vi "main_GBATP_Portain_Sample.vi"() -> ()   [LabVIEW 2020]
panel:
  out "Even Number":dbl=1.0
  out "X, Y, Z, S":i32=3
  out "Value":string="0"
  out "Index 2":i32=95
  out "Index":i32=95
  out "Current Position(mm) 2":dbl
  in  "Occupied Length by Air(mm)  2":dbl format="%#_13g"
  out "Value 2":string="0"
  out "X, Y, Z, S 2":i32=3
  out "Index 4":i32=123
  out "Index 3":i32=123
  in  "Stop Button":bool
  in  "ATP":bool=TRUE
  out "ATP":bool=TRUE
  out "Sample":bool=TRUE
  in  "Occupied Length by Air(mm)  3":dbl format="%#_13g"
  out "Current Position(mm) 3":dbl
  out "ATPPortain":bool=TRUE
  out "X, Y, Z, S 3":i32=3
  out "Index 6":i32=95
  out "Value 3":string="0"
  out "Index 5":i32=95
  in  "Setting Tab":T1(tab)
  out "all rows":string[][](array[string])=[["58"], ["257"], ["0"], ["0"], ["58"], ["257"], ["100"], ["50"], ["58"], ["257"], ["0"], ["50"], ["58"], ["470"], ["0"], ["50"], ["58"], ["470"], ["100"], ["0"], ["58"], ["470"], ["0"], ["0"], ["120"], ["470"], ["0"], ["0"], ["120"], ["470"], ["100"], ["50"], ["120"], ["470"], ["0"], ["50"], ["120"], ["550"], ["0"], ["50"], ["120"], ["550"], ["100"], ["0"], ["120"], ["550"], ["0"], ["0"], ["120"], ["470"], ["0"], ["0"], ["120"], ["470"], ["100"], ["50"], ["120"], ["470"], ["0"], ["50"], ["120"], ["550"], ["0"], ["50"], ["120"], ["550"], ["100"], ["0"], ["120"], ["550"], ["0"], ["0"], ["120"], ["470"], ["0"], ["0"], ["120"], ["470"], ["100"], ["50"], ["120"], ["470"], ["0"], ["50"], ["120"], ["550"], ["0"], ["50"], ["120"], ["550"], ["100"], ["0"], ["120"], ["550"], ["0"], ["0"]]
  in  "format (%.3f)":string="%.3f"
  in  "transpose (no:F)":bool
  in  "type (empty)":string[][](array[string])
  in  "delimiter (Tab)":string="\t"
  out "Size(s)":i32=96
  in  "Sampling Measurement Time(S)":dbl=10.0
  out "Current Position(mm)":dbl
  in  "Occupied Length by Air(mm)":dbl format="%#_13g"
  out "Action":bool=TRUE
  out "Current Time Index":i32=10
  in  "file path (dialog if empty)":path=path "C:/Users/user/Desktop/AutoSampler/AutoSampler _GB/ATP.txt"
  in  "start of read offset (chars.:0)":i32
  in  "max characters/row  (no limit:0)":i32
  out "mark after read (chars.)":i32=406
  in  "number of rows (all:-1)":i32=-1
  out "EOF?":bool
  out "mark after read (chars.) 2":i32=1632
  out "all rows 2":string[][](array[string])=[["58"], ["257"], ["0"], ["0"], ["58"], ["257"], ["100"], ["0"], ["58"], ["257"], ["0"], ["0"], ["58"], ["0"], ["0"], ["0"], ["58"], ["0"], ["100"], ["0"], ["58"], ["0"], ["0"], ["0"], ["120"], ["470"], ["0"], ["0"], ["120"], ["470"], ["100"], ["0"], ["120"], ["470"], ["0"], ["0"], ["120"], ["550"], ["0"], ["0"], ["120"], ["550"], ["100"], ["0"], ["120"], ["550"], ["0"], ["0"], ["120"], ["470"], ["0"], ["0"], ["120"], ["470"], ["100"], ["0"], ["120"], ["470"], ["0"], ["0"], ["120"], ["550"], ["0"], ["0"], ["120"], ["550"], ["100"], ["0"], ["120"], ["550"], ["0"], ["0"], ["120"], ["470"], ["0"], ["0"], ["120"], ["470"], ["100"], ["0"], ["120"], ["470"], ["0"], ["0"], ["120"], ["550"], ["0"], ["0"], ["120"], ["550"], ["100"], ["0"], ["120"], ["550"], ["0"], ["0"], ["58"], ["257"], ["0"], ["0"], ["58"], ["257"], ["100"], ["0"], ["58"], ["257"], ["0"], ["0"], ["58"], ["9"], ["0"], ["0"], ["58"], ["9"], ["100"], ["0"], ["58"], ["9"], ["0"], ["0"], ["120"], ["470"], ["0"], ["0"], ["120"], ["470"], ["100"], ["0"], ["120"], ["470"], ["0"], ["0"], ["120"], ["550"], ["0"], ["0"], ["120"], ["550"], ["100"], ["0"], ["120"], ["550"], ["0"], ["0"], ["120"], ["470"], ["0"], ["0"], ["120"], ["470"], ["100"], ["0"], ["120"], ["470"], ["0"], ["0"], ["120"], ["550"], ["0"], ["0"], ["120"], ["550"], ["100"], ["0"], ["120"], ["550"], ["0"], ["0"]]
  in  "format (%.3f) 2":string="%.3f"
  in  "transpose (no:F) 2":bool
  in  "type (empty) 2":string[][](array[string])
  in  "delimiter (Tab) 2":string="\t"
  out "EOF? 2":bool
  out "Sample Size(s) 2":i32=168
  in  "file path (dialog if empty) 4":path=path "C:/Users/user/Desktop/AutoSampler/AutoSampler _GB/SamplePosition.txt"
  in  "start of read offset (chars.:0) 2":i32
  in  "max characters/row  (no limit:0) 2":i32
  in  "number of rows (all:-1) 2":i32=-1
  in  "file path (dialog if empty) 3":path=path "C:/Users/user/Desktop/AutoSampler/AutoSampler _GB/ProteinPosition.txt"
  out "mark after read (chars.) 3":i32=1632
  out "all rows 3":string[][](array[string])=[["58"], ["63"], ["0"], ["0"], ["58"], ["63"], ["100"], ["0"], ["58"], ["63"], ["0"], ["0"], ["58"], ["257"], ["0"], ["0"], ["58"], ["257"], ["100"], ["0"], ["58"], ["257"], ["0"], ["0"], ["120"], ["470"], ["0"], ["0"], ["120"], ["470"], ["100"], ["0"], ["120"], ["470"], ["0"], ["0"], ["120"], ["550"], ["0"], ["0"], ["120"], ["550"], ["100"], ["0"], ["120"], ["550"], ["0"], ["0"], ["120"], ["470"], ["0"], ["0"], ["120"], ["470"], ["100"], ["0"], ["120"], ["470"], ["0"], ["0"], ["120"], ["550"], ["0"], ["0"], ["120"], ["550"], ["100"], ["0"], ["120"], ["550"], ["0"], ["0"], ["120"], ["470"], ["0"], ["0"], ["120"], ["470"], ["100"], ["0"], ["120"], ["470"], ["0"], ["0"], ["120"], ["550"], ["0"], ["0"], ["120"], ["550"], ["100"], ["0"], ["120"], ["550"], ["0"], ["0"]]
  in  "format (%.3f) 3":string="%.3f"
  in  "transpose (no:F) 3":bool
  in  "type (empty) 3":string[][](array[string])
  in  "delimiter (Tab) 3":string="\t"
  out "EOF? 3":bool
  out "Size(s) 3":i32=96
  in  "start of read offset (chars.:0) 3":i32
  in  "max characters/row  (no limit:0) 3":i32
  in  "number of rows (all:-1) 3":i32=-1
  out "error out":errorcluster={"status"=FALSE, "code"=1073676294, "source"="VISA Read in position_read.vi->main_GBATP_Portain_Sample.vi"}
  out "S Connecting":bool=TRUE
  out "Z Connecting":bool=TRUE
  out "Y Connecting":bool=TRUE
  out "X  Connecting":bool=TRUE
  in  "COM Port":refnum<visa-resource-name>="COM3"
  # "Position :"
  # "(set the Occupied length by Air if the target axis is syringe axis)"
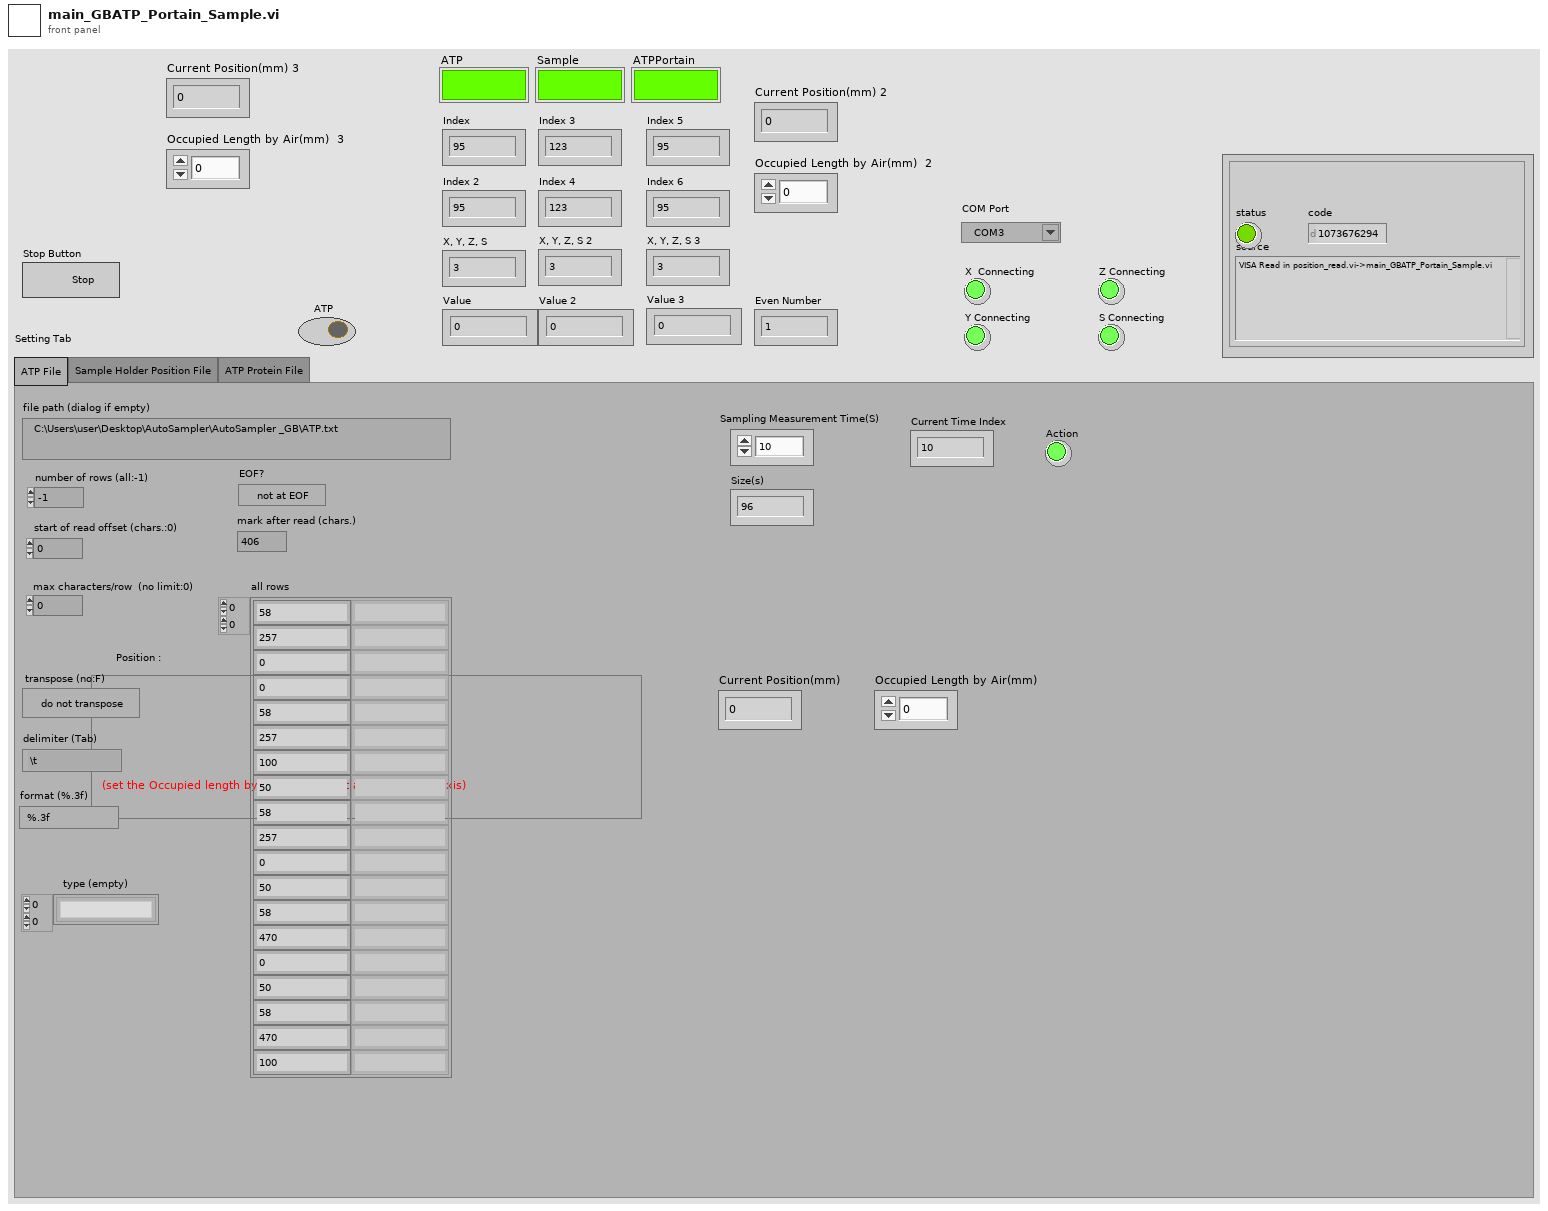
[diagram p1: front panel]
types:
  T1 = enum32{"ATP File", "Sample Holder Position File", "ATP Protein File"}
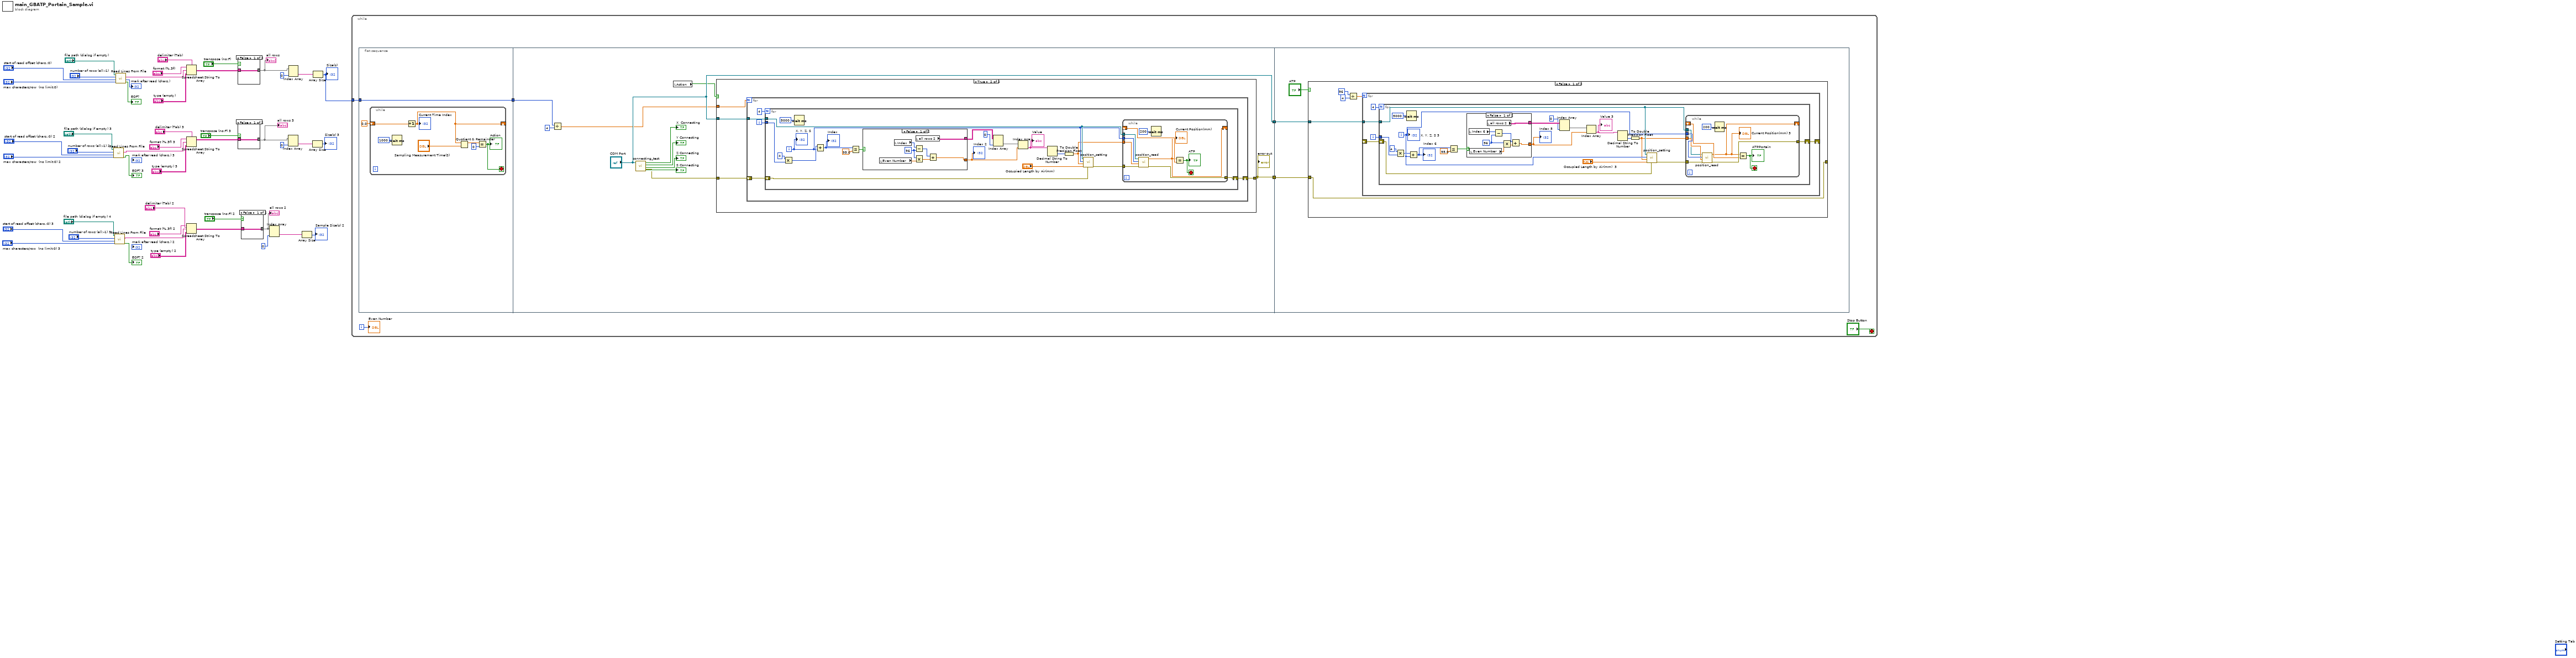
[diagram p0: block diagram]
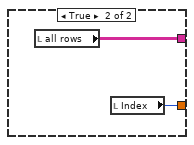
[diagram p3: hidden frame]
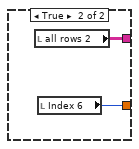
[diagram p4: hidden frame]
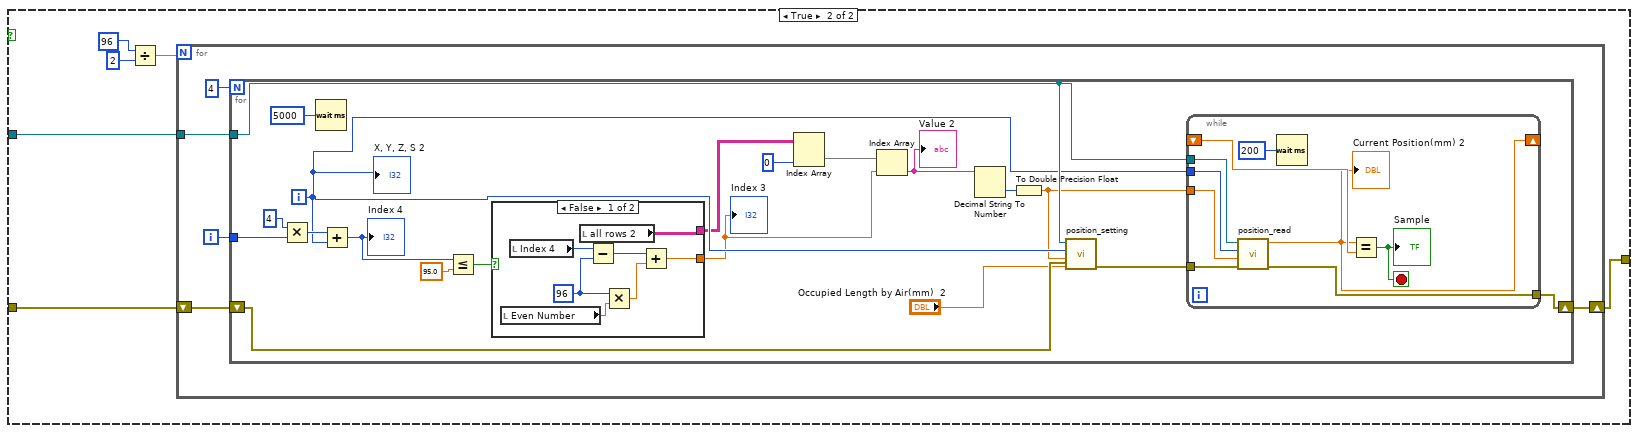
[diagram p5: hidden frame]
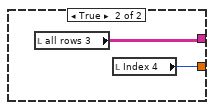
[diagram p6: hidden frame]
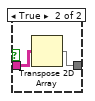
[diagram p7: hidden frame]
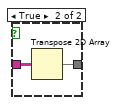
[diagram p8: hidden frame]
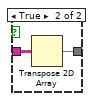
[diagram p9: hidden frame]
diagram:
  n1 = call <vilib>:"Read Lines From File.vi"("file path (dialog if empty)"="file path (dialog if empty) 3", "number of lines (all:-1)"="number of rows (all:-1) 2", "start of read offset (chars.:0)"="start of read offset (chars.:0) 2", "[max characters per line]  (no limit:0)"="max characters/row  (no limit:0) 2") -> ("line string"=w38:string, "EOF?"=→"EOF? 3":bool)  [unwired: 2 in, 2 out]
  n2 = call <vilib>:"Read Lines From File.vi"("file path (dialog if empty)"="file path (dialog if empty) 4", "number of lines (all:-1)"="number of rows (all:-1) 3", "start of read offset (chars.:0)"="start of read offset (chars.:0) 3", "[max characters per line]  (no limit:0)"="max characters/row  (no limit:0) 3") -> ("line string"=w45:string, "EOF?"=→"EOF? 2":bool)  [unwired: 2 in, 2 out]
  n3 = call <vilib>:"Read Lines From File.vi"("file path (dialog if empty)"="file path (dialog if empty)", "number of lines (all:-1)"="number of rows (all:-1)", "start of read offset (chars.:0)"="start of read offset (chars.:0)", "[max characters per line]  (no limit:0)"="max characters/row  (no limit:0)") -> ("line string"=w34:string, "mark after read (chars.)"=→"mark after read (chars.)":i32, "EOF?"=→"EOF?":bool)  [unwired: 2 in, 1 out]
  n4 = Spreadsheet String To Array(delimiter (Tab)="delimiter (Tab)", format string="format (%.3f)", spreadsheet string=w34, array type (2D Dbl)="type (empty)") -> (array=w6:string[][])
  n5 = Spreadsheet String To Array(delimiter (Tab)="delimiter (Tab) 3", format string="format (%.3f) 3", spreadsheet string=w38, array type (2D Dbl)="type (empty) 3") -> (array=w21:string[][])
  n6 = Spreadsheet String To Array(delimiter (Tab)="delimiter (Tab) 2", format string="format (%.3f) 2", spreadsheet string=w45, array type (2D Dbl)="type (empty) 2") -> (array=w12:string[][])
  n7 = case shown="False" "transpose (no:F)" {
    tunnel: [w47 w49] -> w18
    tunnel: w6 -> [w47 w48]
    frame False {
    }
    frame True {
      n8 = Transpose 2D Array(2D array=w48) -> (transposed array=w49:string[][])
    }
  }
  "all rows" <- w18
  n9 = case shown="False" "transpose (no:F) 3" {
    tunnel: [w50 w52] -> w27
    tunnel: w21 -> [w50 w51]
    frame False {
    }
    frame True {
      n10 = Transpose 2D Array(2D array=w51) -> (transposed array=w52:string[][])
    }
  }
  "all rows 3" <- w27
  n11 = case shown="False" "transpose (no:F) 2" {
    tunnel: [w53 w55] -> w19
    tunnel: w12 -> [w53 w54]
    frame False {
    }
    frame True {
      n12 = Transpose 2D Array(2D array=w54) -> (transposed array=w55:string[][])
    }
  }
  "all rows 2" <- w19
  n13 = Index Array "Index Array"(array=w19, index (col)=0) -> (element=w16:string[])  [unwired: 1 in]
  n14 = Index Array "Index Array"(array=w27, index (col)=0) -> (element=w25:string[])  [unwired: 1 in]
  n15 = Index Array "Index Array"(array=w18, index (col)=0) -> (element=w10:string[])  [unwired: 1 in]
  n16 = Array Size(array=w16) -> (size(s)=→"Sample Size(s) 2":i32)
  n17 = Array Size(array=w25) -> (size(s)=→"Size(s) 3":i32)
  n18 = Array Size(array=w10) -> (size(s)=w1:i32)
  "Size(s)" <- w1
  n19 = while {
    tunnel: w1 -> [w58]
    i -> [w56]
    stop <- "Stop Button" stop-if-true
    n20 = flat-sequence {
      tunnel: w58 -> [w63]
      tunnel: [w63] -> w61
      tunnel: [w75] -> w60
      tunnel: ["COM Port"] -> w59
      tunnel: w61 -> [w76]
      tunnel: w60 -> [w130]
      tunnel: w59 -> [w132]
      frame #0 {
        n21 = while {
          shift-right: [w66] -> _
          shift-left: 0.0 ("x") -> [w67]
          stop <- w64 stop-if-true
          n22 = Wait (ms)(milliseconds to wait=u32 1000) -> ()  [unwired: 1 out]
          n23 = Increment(x=w67) -> (x+1=w66:dbl)
          "Current Time Index" <- w66
          n24 = Quotient & Remainder(x=w66, y="Sampling Measurement Time(S)") -> (x-y*floor(x/y)=w70:dbl)  [unwired: 1 out]
          n25 = Equal?(x=w70, y=0) -> (x = y?=w64:bool)
          "Action" <- w64
        }
      }
      frame #1 {
        n26 = Divide(x=w76, y=4) -> (x/y=w72:dbl)
        n27 = call "connecting_test.vi"("VISA resource name"="COM Port") -> ("syringe axis connecting"=→"S Connecting":bool, "Z axis connecting"=→"Z Connecting":bool, "Y axis connecting"=→"Y Connecting":bool, "X axis connecting"=→"X  Connecting":bool, "error out"=w78:errorcluster)  [unwired: 6 in]
        n28 = local read "Action"() -> (w71:bool)
        n29 = case shown="True" w71 {
          tunnel: w78 -> [w82 w86]
          tunnel: [w82 w85] -> w75
          tunnel: "COM Port" -> [_ w84]
          tunnel: w72 -> [_ w83]
          frame False {
          }
          frame True {
            n30 = for {
              N: w83 -> [_]
              tunnel: w84 -> [w89]
              shift-right: [w90] -> w85
              shift-left: w86 -> [w91]
              i -> [w87]
              n31 = for {
                N: 4 -> [_]
                tunnel: w89 -> [w107]
                shift-right: [w110] -> w90
                shift-left: w91 -> [w111]
                tunnel: w87 -> [w96]
                i -> [w104]
                n32 = Multiply(x=4, y=w96) -> (x*y=w106:i32)
                n33 = Wait (ms)(milliseconds to wait=u32 5000) -> ()  [unwired: 1 out]
                n34 = Add(x=w106, y=w104) -> (x+y=w93:i32)
                "Index" <- w93
                n35 = Less Or Equal?(x=w93, y=95.0) -> (x <= y?=w95:bool)
                n36 = case shown="False" w95 {
                  tunnel: [w118 w120] -> w102
                  tunnel: [w113 w119] -> w92
                  frame False {
                    w116 = 96 ("y")
                    n37 = local read "Even Number"() -> (w112:dbl)
                    n38 = local read "Index"() -> (w117:i32)
                    n39 = Subtract(x=w117, y=w116) -> (x-y=w115:i32)
                    n40 = Multiply(x=w116, y=w112) -> (x*y=w114:dbl)
                    n41 = local read "all rows 2"() -> (w118:string[][])
                    n42 = Add(x=w115, y=w114) -> (x+y=w113:dbl)
                  }
                  frame True {
                    n43 = local read "all rows"() -> (w120:string[][])
                    n44 = local read "Index"() -> (w119:i32)
                  }
                }
                "Index 2" <- w92
                n45 = Index Array "Index Array"(array=w102, index (col)=0) -> (element=w103:string[])  [unwired: 1 in]
                n46 = Index Array(array=w103, index=w92) -> (element=w100:string)
                "Value" <- w100
                n47 = Decimal String To Number(string=w100) -> (number=w98:i32)  [unwired: 2 in, 1 out]
                n48 = To Double Precision Float(number=w98) -> (double precision float=w97:dbl)
                n49 = call "position_setting.vi"("error in (no error)"=w111, "Occupied length by Air(mm)"="Occupied Length by Air(mm)", "Distance(mm)"=w97, "Axis"=w104, "Com Port"=w107) -> ("error out"=w109:errorcluster)  [unwired: 6 in]
                n50 = while {
                  tunnel: w104 -> [w129]
                  tunnel: w97 -> [w128]
                  tunnel: [w127] -> w110
                  tunnel: w109 -> [w126]
                  shift-right: [w124] -> _
                  shift-left: _ -> [w125]
                  tunnel: w107 -> [w121]
                  stop <- w122 stop-if-true
                  n51 = call "position_read.vi"("error in (no error)"=w126, "Occupied Length by Air(mm)"=w128, "Axis"=w129, "COM Port"=w121) -> ("error out"=w127:errorcluster, "current position(mm)"=w124:dbl)  [unwired: 6 in]
                  "Current Position(mm)" <- w124
                  n52 = Wait (ms)(milliseconds to wait=u32 200) -> ()  [unwired: 1 out]
                  n53 = Equal?(x=w124, y=w125) -> (x = y?=w122:bool)
                  "ATP" <- w122
                }
                "X, Y, Z, S" <- w104
              }
            }
          }
        }
        "error out" <- w75
      }
      frame #2 {
        n54 = case shown="False" "ATP" {
          tunnel: w130 -> [w137 w186]
          tunnel: [w137 w185] -> _
          tunnel: w132 -> [w136 w184]
          frame False {
            n55 = Divide(x=96, y=4) -> (x/y=w133:dbl)
            n56 = for {
              N: w133 -> [_]
              tunnel: w136 -> [w140]
              shift-right: [w141] -> _
              shift-left: _ -> [w142]
              i -> [w138]
              n57 = for {
                N: 4 -> [_]
                tunnel: w140 -> [w158]
                shift-right: [w161] -> w141
                shift-left: w142 -> [w162]
                tunnel: w138 -> [w147]
                i -> [w155]
                n58 = Multiply(x=4, y=w147) -> (x*y=w157:i32)
                n59 = Wait (ms)(milliseconds to wait=u32 5000) -> ()  [unwired: 1 out]
                n60 = Add(x=w157, y=w155) -> (x+y=w144:i32)
                "Index 6" <- w144
                n61 = Less Or Equal?(x=w144, y=95.0) -> (x <= y?=w146:bool)
                n62 = case shown="False" w146 {
                  tunnel: [w164 w170] -> w153
                  tunnel: [w165 w171] -> w143
                  frame False {
                    w168 = 96 ("y")
                    n63 = local read "Index 6"() -> (w169:i32)
                    n64 = local read "Even Number"() -> (w163:dbl)
                    n65 = local read "all rows 2"() -> (w164:string[][])
                    n66 = Subtract(x=w169, y=w168) -> (x-y=w167:i32)
                    n67 = Multiply(x=w168, y=w163) -> (x*y=w166:dbl)
                    n68 = Add(x=w167, y=w166) -> (x+y=w165:dbl)
                  }
                  frame True {
                    n69 = local read "all rows 2"() -> (w170:string[][])
                    n70 = local read "Index 6"() -> (w171:i32)
                  }
                }
                "Index 5" <- w143
                n71 = Index Array "Index Array"(array=w153, index (col)=0) -> (element=w154:string[])  [unwired: 1 in]
                n72 = Index Array(array=w154, index=w143) -> (element=w151:string)
                "Value 3" <- w151
                n73 = Decimal String To Number(string=w151) -> (number=w149:i32)  [unwired: 2 in, 1 out]
                n74 = To Double Precision Float(number=w149) -> (double precision float=w148:dbl)
                n75 = call "position_setting.vi"("error in (no error)"=w162, "Occupied length by Air(mm)"="Occupied Length by Air(mm)  3", "Distance(mm)"=w148, "Axis"=w155, "Com Port"=w158) -> ("error out"=w160:errorcluster)  [unwired: 6 in]
                n76 = while {
                  tunnel: w155 -> [w180]
                  tunnel: w148 -> [w179]
                  tunnel: [w178] -> w161
                  tunnel: w160 -> [w177]
                  shift-right: [w175] -> _
                  shift-left: _ -> [w176]
                  tunnel: w158 -> [w172]
                  stop <- w173 stop-if-true
                  n77 = call "position_read.vi"("error in (no error)"=w177, "Occupied Length by Air(mm)"=w179, "Axis"=w180, "COM Port"=w172) -> ("error out"=w178:errorcluster, "current position(mm)"=w175:dbl)  [unwired: 6 in]
                  "Current Position(mm) 3" <- w175
                  n78 = Wait (ms)(milliseconds to wait=u32 200) -> ()  [unwired: 1 out]
                  n79 = Equal?(x=w175, y=w176) -> (x = y?=w173:bool)
                  "ATPPortain" <- w173
                }
                "X, Y, Z, S 3" <- w155
              }
            }
          }
          frame True {
            n80 = Divide(x=96, y=2) -> (x/y=w181:dbl)
            n81 = for {
              N: w181 -> [_]
              tunnel: w184 -> [w189]
              shift-right: [w190] -> w185
              shift-left: w186 -> [w191]
              i -> [w187]
              n82 = for {
                N: 4 -> [_]
                tunnel: w189 -> [w207]
                shift-right: [w210] -> w190
                shift-left: w191 -> [w211]
                tunnel: w187 -> [w196]
                i -> [w204]
                n83 = Multiply(x=4, y=w196) -> (x*y=w206:i32)
                n84 = Wait (ms)(milliseconds to wait=u32 5000) -> ()  [unwired: 1 out]
                n85 = Add(x=w206, y=w204) -> (x+y=w193:i32)
                "Index 4" <- w193
                n86 = Less Or Equal?(x=w193, y=95.0) -> (x <= y?=w195:bool)
                n87 = case shown="False" w195 {
                  tunnel: [w213 w219] -> w202
                  tunnel: [w214 w220] -> w192
                  frame False {
                    w217 = 96 ("y")
                    n88 = local read "Even Number"() -> (w212:dbl)
                    n89 = local read "Index 4"() -> (w218:i32)
                    n90 = local read "all rows 2"() -> (w213:string[][])
                    n91 = Subtract(x=w218, y=w217) -> (x-y=w216:i32)
                    n92 = Multiply(x=w217, y=w212) -> (x*y=w215:dbl)
                    n93 = Add(x=w216, y=w215) -> (x+y=w214:dbl)
                  }
                  frame True {
                    n94 = local read "all rows 3"() -> (w219:string[][])
                    n95 = local read "Index 4"() -> (w220:i32)
                  }
                }
                "Index 3" <- w192
                n96 = Index Array "Index Array"(array=w202, index (col)=0) -> (element=w203:string[])  [unwired: 1 in]
                n97 = Index Array(array=w203, index=w192) -> (element=w200:string)
                "Value 2" <- w200
                n98 = Decimal String To Number(string=w200) -> (number=w198:i32)  [unwired: 2 in, 1 out]
                n99 = To Double Precision Float(number=w198) -> (double precision float=w197:dbl)
                n100 = call "position_setting.vi"("error in (no error)"=w211, "Occupied length by Air(mm)"="Occupied Length by Air(mm)  2", "Distance(mm)"=w197, "Axis"=w204, "Com Port"=w207) -> ("error out"=w209:errorcluster)  [unwired: 6 in]
                n101 = while {
                  tunnel: w204 -> [w229]
                  tunnel: w197 -> [w228]
                  tunnel: [w227] -> w210
                  tunnel: w209 -> [w226]
                  shift-right: [w224] -> _
                  shift-left: _ -> [w225]
                  tunnel: w207 -> [w221]
                  stop <- w222 stop-if-true
                  n102 = call "position_read.vi"("error in (no error)"=w226, "Occupied Length by Air(mm)"=w228, "Axis"=w229, "COM Port"=w221) -> ("error out"=w227:errorcluster, "current position(mm)"=w224:dbl)  [unwired: 6 in]
                  "Current Position(mm) 2" <- w224
                  n103 = Wait (ms)(milliseconds to wait=u32 200) -> ()  [unwired: 1 out]
                  n104 = Equal?(x=w224, y=w225) -> (x = y?=w222:bool)
                  "Sample" <- w222
                }
                "X, Y, Z, S 2" <- w204
              }
            }
          }
        }
      }
    }
    "Even Number" <- w56
  }
